vi "Configure Trace Type.vi"(8 "error in (no error)":errorcluster {"code" format="%.0x"}, 9 "trace type (Clear Write)":i32(ring)=1 items=["Clear Write"=1, "Maximum Hold"=2, "Minimum Hold"=3, "Video Average"=4, "View"=5, "Store"=6], 10 "trace name":string="Trace1" caption="trace name (Trace1)", 11 "instrument handle":refnum<k15>) -> (0 "error out":errorcluster {"code" format="%.0x"}, 3 "instrument handle out":refnum<k15>)   [LabVIEW 2009, in "Keysight XSAn.lvlib"]
doc: "This VI configures the Trace Type property.\n\nSupported Models: M9290A, N8973B, N8974B, N8975B, N8976B, N9000A, N9000B, N9010A, N9010B, N9020A, N9020B, N9030A, N9030B, N9038A, N9040B, N9041B, SPN9003A, SPN9026A"
uses:
  <instrlib>/Keysight XSAn/Keysight XSAn.lvlib
  AgXSAn.dll
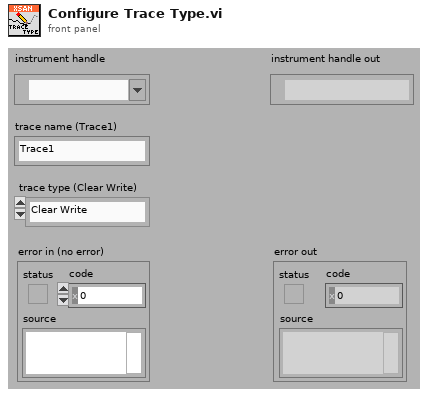
[diagram p1: front panel]
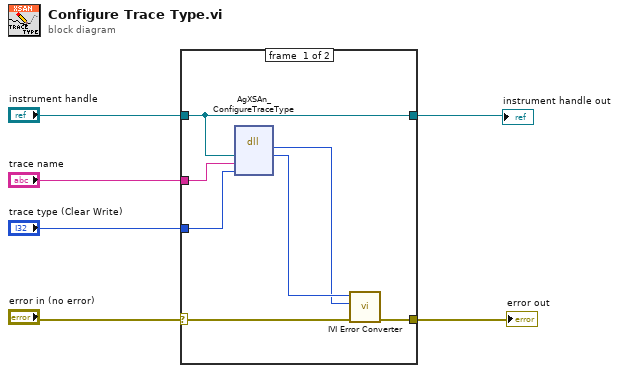
[diagram p0: block diagram]
diagram:
  n1 = case shown="No Error" "error in (no error)" {
    selector: "error in (no error)" -> [w11 w15]
    tunnel: "instrument handle" -> [w9 w14]
    tunnel: [w12 w15] -> w4
    tunnel: [w9 w14] -> w3
    tunnel: "trace name" -> [w8 _]
    tunnel: "trace type (Clear Write)" -> [w7 _]
    frame #0 {
      n2 = dll-call lib="AgXSAn**.dll" fn="AgXSAn_ConfigureTraceType" ("LabVIEW:IviSpecAn_ConfigureTraceType")("instrument handle"=w9, "trace name"=w8, "trace type"=w7) -> ("Status"=w10:i32, "instrument handle"=w13:u32)  [unwired: 5 in, 2 out]
      n3 = call <instrlib>:"IVI Error Converter.vi"("error in (no error)"=w11, "IVI error code (0)"=w10, "instrument handle"=w13) -> ("error out"=w12:errorcluster)  [unwired: 7 in, 1 out]
    }
    frame #1 {
    }
  }
  "error out" <- w4
  "instrument handle out" <- w3
